vi "data-logging-example.vi"() -> ()   [LabVIEW 2023]
panel:
  out "keep file open?":bool=TRUE
  in  "Datalogging options":T1={"Include Timestamp"=TRUE, "Include milliseconds"=FALSE, "data-precision"=3}
  in  "Log Filepath Source":T2(ring)
  in  "Log File Folder Name":string="data"
  out "Logged CSV out":string
  in  "format array to string":string="%.2f"
  out "array input":dbl[](array[numeric])
  out "Running":bool
  in  "CSV Data Headings":string="timestamp, data1, data2, data3, data4,"
  in  "Include Seconds in Filename":bool
  in  "Include Date in Filename":bool=TRUE
  in  "Include Time in Filename":bool=TRUE
  out "iteration":i32
  out "data4":dbl format="%.2f"
  out "data3":dbl format="%.2f"
  out "data2":dbl format="%.2f"
  out "data1":dbl format="%.2f"
  out "date string":string
  out "time string":string
  in  "log file name":string="log"
  out "Log File Path":path
  out "error IO":errorcluster
  in  "Log File Path (Manual)":path=path "data"
  in  "Start":bool
  # "File Naming Options"
  # "Data Being Written"
  # "File Contents Options"
  # "Warning: If using mS -> Excel will not display as time format - cells can be manually changed to display correct format\nor open as text file."
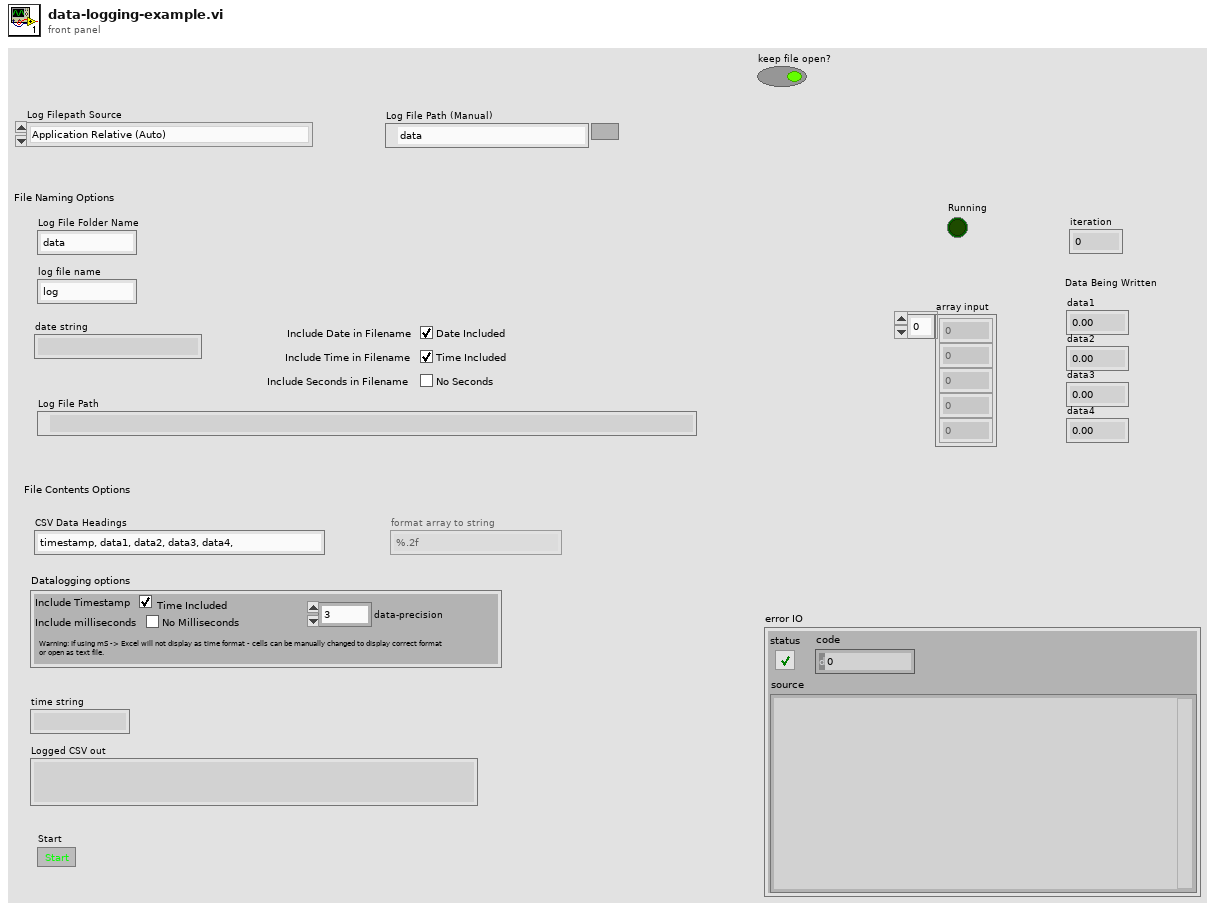
[diagram p1: front panel]
types:
  T1 = cluster{"Include Timestamp":bool, "Include milliseconds":bool, "data-precision":i32}
  T2 = enum16{"Application Relative (Auto)", "VI Relative (Auto)", "Complete Path (Manual)"}
  T3 = enum8{"Enabled", "Disabled", "Disabled and Grayed Out"}
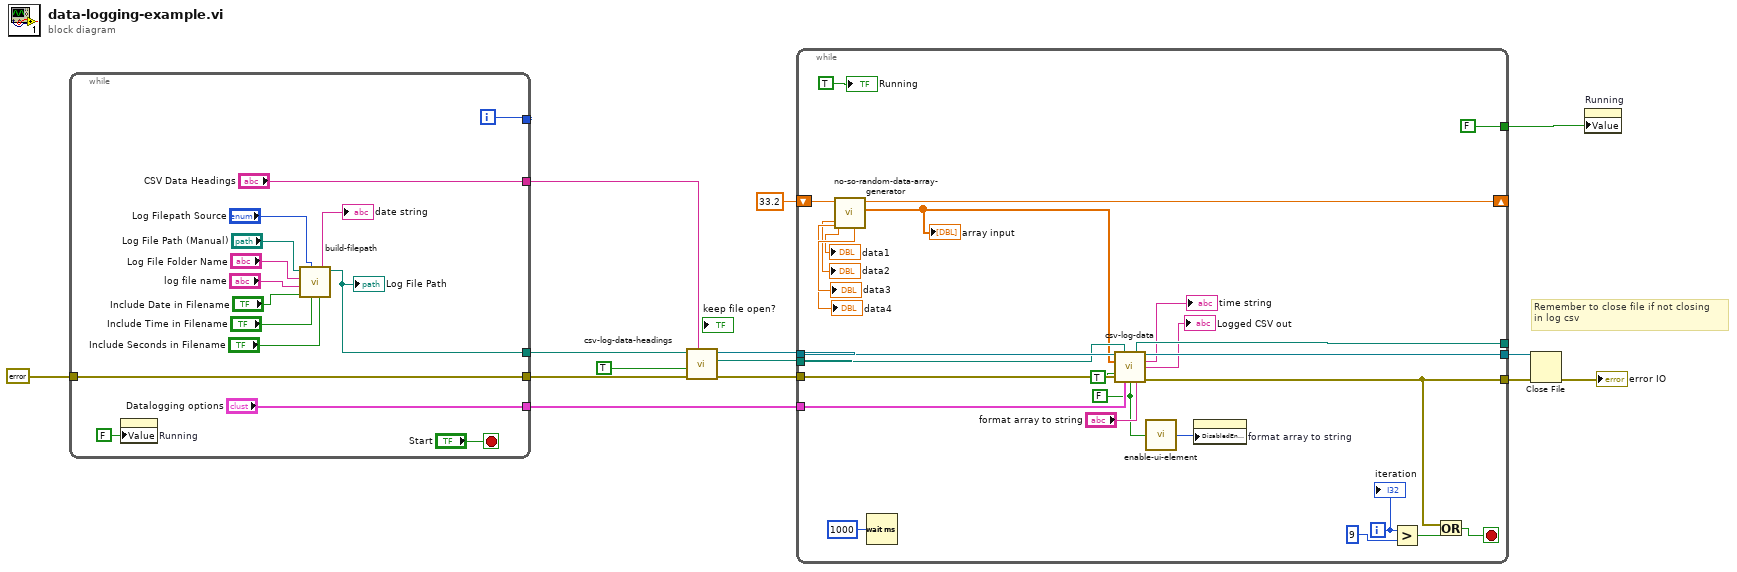
[diagram p0: block diagram]
diagram:
  # "Remember to close file if not closing\nin log csv"
  n1 = while {
    tunnel: [w28] -> w13
    tunnel: errorcluster {"status"=FALSE, "code"=0, "source"=""} ("error in") -> [w28]
    tunnel: [w27] -> _
    tunnel: [w25] -> w8
    tunnel: ["Datalogging options"] -> w6
    tunnel: ["CSV Data Headings"] -> w1
    i -> [w27]
    stop <- "Start" stop-if-true
    n2 = property on="Running" class="Bool (strict)"("Value"=FALSE ("Running")) -> ()  [unwired: 2 in, 2 out]
    n3 = call "build-filepath.vi"("Include Seconds in Filename"="Include Seconds in Filename", "Include Time in Filename"="Include Time in Filename", "Log Filepath Source"="Log Filepath Source", "Include Date in Filename"="Include Date in Filename", "log file name"="log file name", "Log File Folder Name"="Log File Folder Name", "Log File Path"="Log File Path (Manual)") -> ("appended path for log file"=w25:path, "date string"=→"date string":string)  [unwired: 3 in]
    "Log File Path" <- w25
  }
  n4 = call "csv-log-data-headings.vi"("CSV Data Headings"=w1, "error in (no error)"=w13, "keep file open?"=TRUE, "Log File Path"=w8) -> ("error out"=w11:errorcluster, "Log File Path"=w5:path, "Byte Stream File out"=w12:refnum<file>)  [unwired: 5 in]
  n5 = while {
    tunnel: w12 -> [w44]
    tunnel: w11 -> [w45]
    shift-right: [w50] -> _
    shift-left: 33.2 -> [w51]
    tunnel: w6 -> [w39]
    tunnel: w5 -> [w42]
    tunnel: [w33] -> w4
    tunnel: [w43] -> w3
    tunnel: [w41] -> _
    tunnel: [FALSE ("Running")] -> w2
    i -> [w56]
    stop <- w53 stop-if-true
    w35 = FALSE ("Override Format Array?")
    n6 = call "no-so-random-data-array-generator.vi"("Numeric in"=w51) -> ("data4"=→"data4":dbl, "Array Out"=w32:dbl[], "Numeric out"=w50:dbl, "data3"=→"data3":dbl, "data2"=→"data2":dbl, "data1"=→"data1":dbl)  [unwired: 5 in]
    "array input" <- w32
    n7 = Wait (ms)(milliseconds to wait=u32 1000) -> ()  [unwired: 1 out]
    n8 = call "csv-log-data.vi"("log file Byte Stream File in"=w44, "log file path"=w42, "Data Array In"=w32, "File Open?"=TRUE, "error in (no error)"=w45, "Datalogging options"=w39, "Override Format Array?"=w35, "Format Array Override"="format array to string") -> ("log file path"=w41:path, "log file Byte Stream File out"=w43:refnum<file>, "time string"=→"time string":string, "Logged CSV out"=→"Logged CSV out":string, "error out"=w33:errorcluster)  [unwired: 3 in]
    n9 = call "enable-ui-element.vi"("Enable UI Element"=w35) -> ("UI Element State"=w34:T3)  [unwired: 8 in]
    n10 = property on="format array to string" class="Str"("DisabledEnum"=w34) -> ()  [unwired: 2 in, 2 out]
    n11 = Greater?(x=w56, y=9) -> (0:w54:bool)
    n12 = Or(x=w33, y=w54) -> (x .or. y?=w53:bool)
    "iteration" <- w56
    "Running" <- TRUE ("Running")
  }
  n13 = Close File(refnum=w3, error in=w4) -> (error out=→"error IO":errorcluster)  [unwired: 1 out]
  n14 = property on="Running" class="Bool (strict)"("Value"=w2) -> ()  [unwired: 2 in, 2 out]
